vi "Find Windows.vi"(8 "error in (no error)":errorcluster, 11 "VI reference":refnum<vi>) -> (0 "error out":errorcluster, 3 "hWnd":u32)   [LabVIEW 2019, in "Test Bench Tools.lvlib"]
uses:
  Test Bench Tools.lvlib
  user32.dll
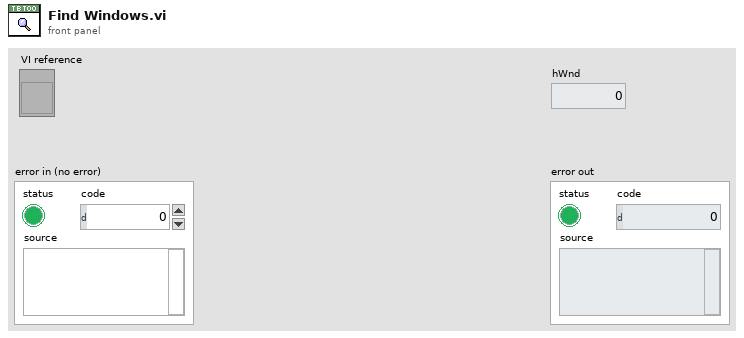
[diagram p1: front panel]
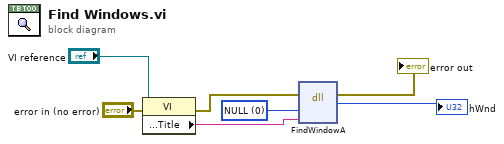
[diagram p0: block diagram]
diagram:
  w6 = 0 items=["NULL"]
  n1 = property class="VI"(reference="VI reference", error in="error in (no error)") -> (error out=w5:errorcluster, "Front Panel.Title"=w7:string)  [unwired: 1 out]
  n2 = dll-call lib="user32.dll" fn="FindWindowA" label="FindWindow"(error in=w5, "lpszClassName"=w6, "lpszWindowName"=w7) -> (error out=→"error out":errorcluster, "hWnd"=→"hWnd":u32)  [unwired: 4 in, 1 out]
